vi "Save Data.vi"(8 "error in (no error)":errorcluster, 11 "Tektronix Driver in":refnum<class "Tektronix 7000 Driver.lvclass">) -> (0 "error out":errorcluster, 1 "Finished":bool, 2 "Current read position":i32, 3 "Tektronix Driver out":refnum<class "Tektronix 7000 Driver.lvclass">)   [LabVIEW 2020, in "Tektronix 7000 Driver.lvclass"]
uses:
  Tektronix 7000 Driver.lvclass
  C:/GitHub/NHMFL_Core/Libraries/Instruments/Pulse Driver/Pulse Driver.lvclass
  C:/GitHub/NHMFL_Core/Libraries/Instruments/Instrument Driver/Instrument Driver.lvclass
  Pulse Driver/Pulse Driver.lvclass/Pulse Driver.ctl
  Pulse Driver/Read tdms file.vi
  Pulse Driver/Write tdms file.vi
  <vilib>/Waveform/WDTOps.llb/WDT Number of Waveform Samples DBL.vi
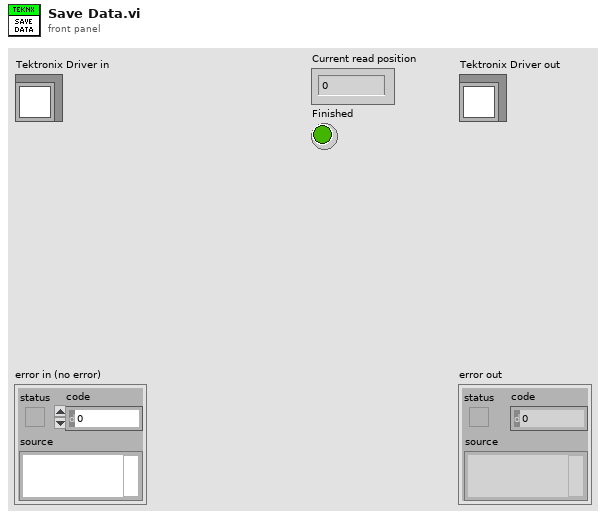
[diagram p1: front panel]
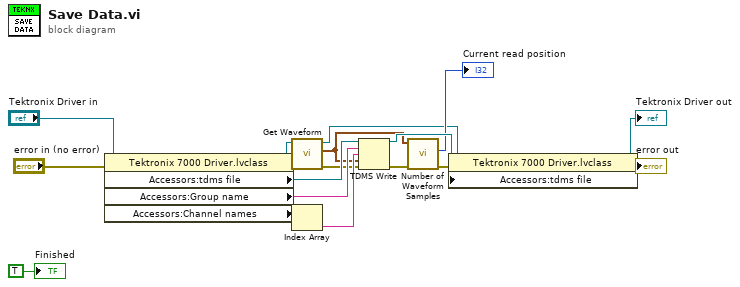
[diagram p0: block diagram]
diagram:
  n1 = property class="Tektronix 7000 Driver.lvclass"(reference="Tektronix Driver in", error in="error in (no error)") -> (reference out=w5:refnum<class "Tektronix 7000 Driver.lvclass">, error out=w3:errorcluster, "Accessors:tdms file"=w16:refnum<k34>, "Accessors:Group name"=w15:string, "Accessors:Channel names"=w14:string[])
  n2 = call-dynamic "Get Waveform.vi"("error in (no error)"=w3, "Tektronix Driver in"=w5) -> ("error out"=w2:errorcluster, "Waveform"=w1:waveform(dbl), "Tektronix Driver out"=w4:refnum<class "Tektronix 7000 Driver.lvclass">)  [unwired: 7 in]
  n3 = Index Array(array=w14) -> (element=w13:string)  [unwired: 1 in]
  n4 = TDMS Write(0:w16, 5:w15, 7:w13, 9:w1, 11:w2) -> (4:w12:refnum<k34>, 15:w8:errorcluster)  [unwired: 1 in, 2 out]
  n5 = call-poly <vilib>:"Number of Waveform Samples.vi"("error in (no error)"=w8, "waveform in"=w1) -> ("error out"=w7:errorcluster, "number of samples"=→"Current read position":i32)  [unwired: 7 in, 1 out]
  n6 = property class="Tektronix 7000 Driver.lvclass"(reference=w4, error in=w7, "Accessors:tdms file"=w12) -> (reference out=→"Tektronix Driver out":refnum<class "Tektronix 7000 Driver.lvclass">, error out=→"error out":errorcluster)
  "Finished" <- TRUE ("Finished")
